vi "rozklad_wielomianu.vi"(8 "x0":dbl, 9 "c":dbl, 10 "b":dbl, 11 "a":dbl) -> (1 "cp":dbl, 2 "bp":dbl, 3 "ap":dbl)   [LabVIEW 2020]
doc: "rozkład wielomianu"
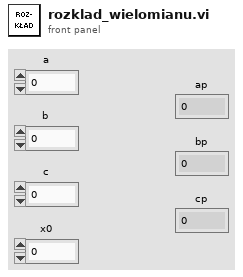
[diagram p1: front panel]
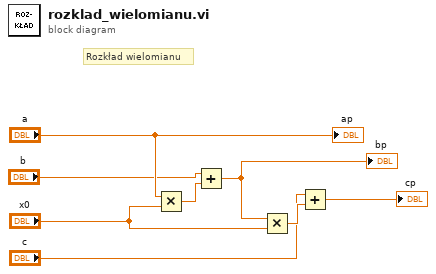
[diagram p0: block diagram]
diagram:
  # "Rozkład wielomianu"
  n1 = Multiply(x="a", y="x0") -> (x*y=w5:dbl)
  n2 = Add(x="b", y=w5) -> (x+y=w6:dbl)
  "bp" <- w6
  n3 = Multiply(x=w6, y="x0") -> (x*y=w8:dbl)
  n4 = Add(x="c", y=w8) -> (x+y=→"cp":dbl)
  "ap" <- "a"
